vi "Frequency.vi"   [LabVIEW 2013, in "NI_EP_Basic.lvlib"]
doc: "Calculates the fundamental frequency of a voltage or current signal. Wire data to the <B>waveform</B> input to determine the polymorphic instance to use or manually select the instance."
uses:
  <vilib>/addons/Electrical Power/Basic/NI_EP_Basic.lvlib
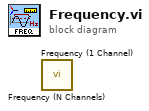
[diagram p0: block diagram]
diagram:
  n1 = call <vilib>:"Frequency (N Channels).vi"() -> ()  [unwired: 10 in, 2 out]
  n2 = call <vilib>:"Frequency (1 Channel).vi"() -> ()  [unwired: 10 in, 2 out]
